vi "数据插入.vi"(5 "数据标记表":string(combo)="N", 7 "测量模式":string(combo), 8 "error in (no error)":errorcluster caption="错误输入（无错误）", 10 "data in":T1={"因子编码"="", "单位"="", "标样参考值"=0.0, "水样数据时间"=timestamp(0 s since 1904-01-01), "水样实测值"=0.0, "水样数据标识"="N", "探头温度"=0.0}, 11 "table输入":string(combo)) -> (0 "error out":errorcluster caption="错误输出")   [LabVIEW 2016, in "斯坦道多参数.lvlib"]
uses:
  <vilib>/Utility/sysdir.llb/System Directory Type.ctl
  <vilib>/addons/database/Connection.llb/DB Tools Open Connec (String).vi
  <vilib>/addons/database/NI_Database_API.lvlib
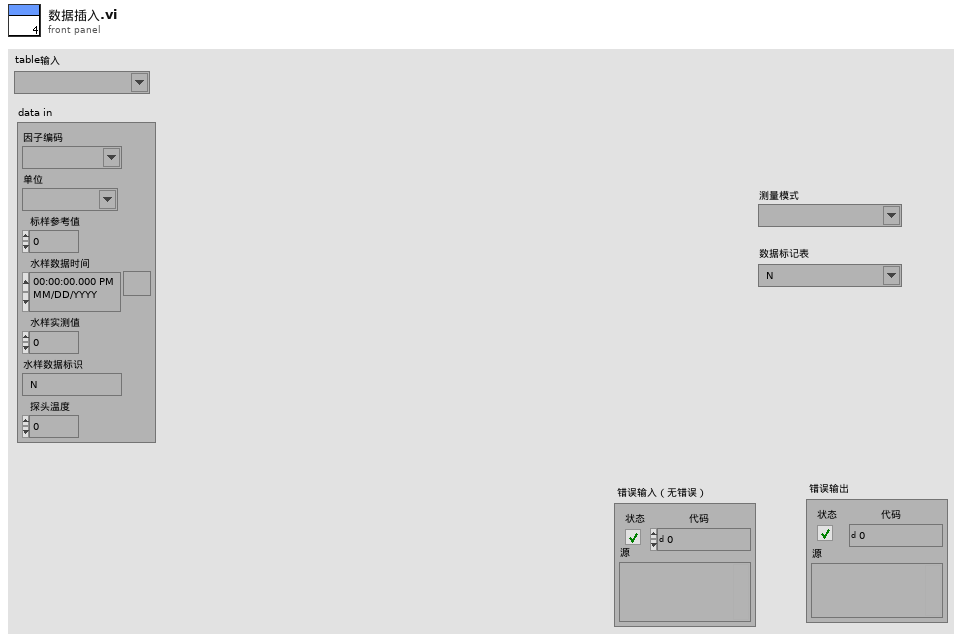
[diagram p1: front panel]
types:
  T1 = cluster{"因子编码":string, "单位":string, "标样参考值":sgl, "水样数据时间":timestamp, "水样实测值":sgl, "水样数据标识":string, "探头温度":sgl}
  T2 = typedef "System Directory Type.ctl" = i32
  T3 = cluster{"时间标识":timestamp, "测量模式":string, "数据类型":string, "监测值":sgl, "单位":string, "数据标识":string, "因子编码":string, "标样参考值":sgl, "探头温度":sgl}
  T4 = typedef "NI_Database_API.lvlib/Conn ObjectReference.ctl" = refnum<k1>
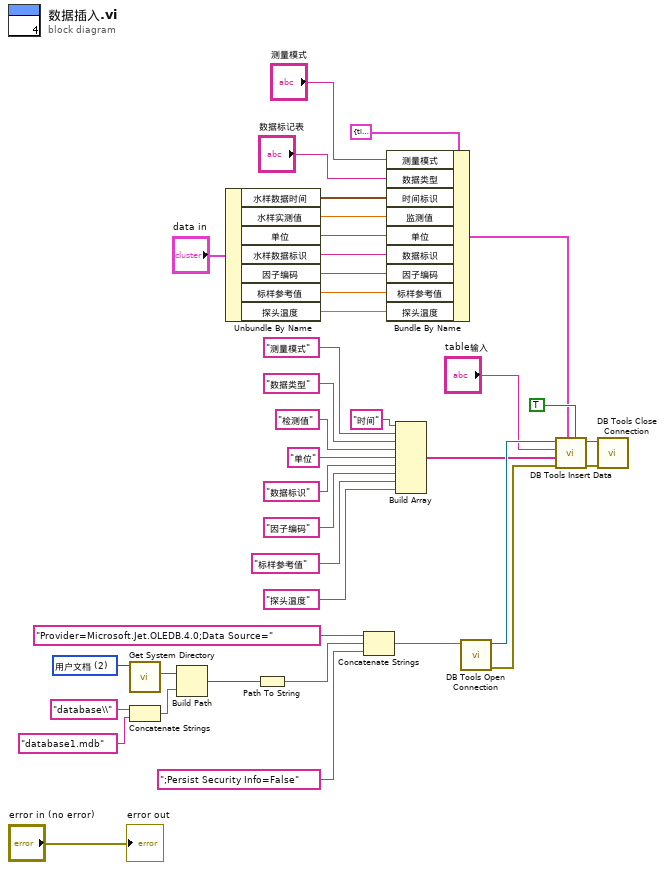
[diagram p0: block diagram]
diagram:
  w20 = T2 2 items=["用户目录"=0, "用户桌面"=1, "用户文档"=2, "用户应用程序数据"=3, "用户设置"=4, "用户临时目录"=5, "公共文档"=6, "公共应用程序数据"=7, "公共设置"=8, "公共缓存"=13, "系统核心库"=9, "系统安装库"=10, "应用程序文件"=11, "启动盘根目录"=12] ("system directory type")
  n1 = call <vilib>:"Get System Directory.vi"("system directory type"=w20) -> ("system directory"=w18:path)  [unwired: 10 in]
  n2 = Concatenate Strings("database\\" ("condition"), "database1.mdb" ("字符串")) -> (w12:string)
  n3 = Build Path(base path=w18, name or relative path=w12) -> (appended path=w17:path)
  n4 = Unbundle By Name("data in") -> ("水样数据时间"=w34:timestamp, "水样实测值"=w33:sgl, "单位"=w29:string, "水样数据标识"=w32:string, "因子编码"=w28:string, "标样参考值"=w30:sgl, "探头温度"=w6:sgl)
  n5 = Path To String(path=w17) -> (string=w16:string)
  n6 = Concatenate Strings("Provider=Microsoft.Jet.OLEDB.4.0;Data Source=" ("condition"), w16, ";Persist Security Info=False" ("condition")) -> (w14:string)
  n7 = Bundle By Name(cluster=T3 {"时间标识"=timestamp(0 s since 1904-01-01), "测量模式"="", "数据类型"="", "监测值"=0.0, "单位"="", "数据标识"="", "因子编码"="", "标样参考值"=0.0, "探头温度"=0.0} ("data输出"), "测量模式"="测量模式", "数据类型"="数据标记表", "时间标识"=w34, "监测值"=w33, "单位"=w29, "数据标识"=w32, "因子编码"=w28, "标样参考值"=w30, "探头温度"=w6) -> (w8:T3)
  n8 = Build Array("时间", "测量模式", "数据类型", "检测值", "单位", "数据标识", "因子编码", "标样参考值", "探头温度") -> (w9:string[])
  n9 = call-poly <vilib>:"DB Tools Open Connection.vi"("connection information"=w14) -> ("error out"=w10:errorcluster, "connection reference"=w11:T4)  [unwired: 7 in]
  n10 = call <vilib>:"DB Tools Insert Data.vi"("create table? (F)"=TRUE, "data"=w8, "error in (no error)"=w10, "columns"=w9, "table"="table输入", "connection reference"=w11) -> ("error out"=w22:errorcluster, "connection reference out"=w23:T4)  [unwired: 4 in]
  n11 = call <vilib>:"DB Tools Close Connection.vi"("error in (no error)"=w22, "connection reference"=w23) -> ()  [unwired: 5 in, 1 out]
  "error out" <- "error in (no error)"
